vi "ALTS-2015 LV2GBL Login Status.vi"(6 "Options":T1=enum."Set", 8 "error in (no error)":errorcluster, 11 "Login Status?":bool) -> (0 "error out":errorcluster, 3 "Login Status?":bool)   [LabVIEW 2013]
uses:
  Controls/ALTS-2015 LV2 Options.ctl
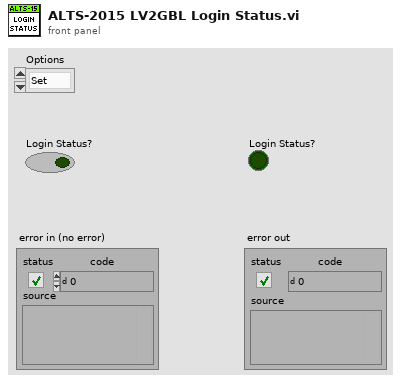
[diagram p1: front panel]
types:
  T1 = typedef "ALTS-2015 LV2 Options.ctl" = enum16{"Get", "Set"}
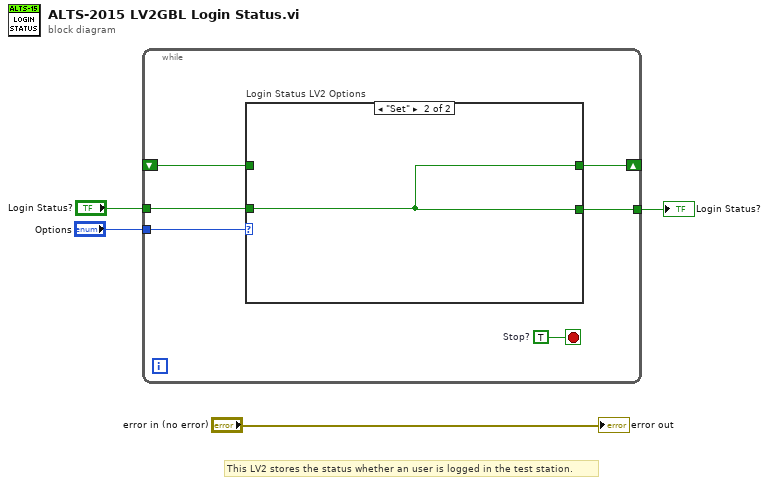
[diagram p0: block diagram]
diagram:
  # "This LV2 stores the status whether an user is logged in the test station."
  n1 = while {
    tunnel: "Options" -> [w10]
    shift-right: [w8] -> _
    shift-left: _ -> [w6]
    tunnel: "Login Status?" -> [w9]
    tunnel: [w7] -> w2
    stop <- w5 stop-if-true
    w5 = TRUE  # Stop?
    n2 = case "Login Status LV2 Options" shown="\"Set\"" w10 {
      tunnel: w9 -> [_ w12]
      tunnel: [w11 w12] -> w8
      tunnel: [w11 w12] -> w7
      tunnel: w6 -> [w11 _]
      frame "Get", Default {
      }
      frame "Set" {
      }
    }
  }
  "Login Status?" <- w2
  "error out" <- "error in (no error)"
